vi "Esis_PitchRollAng_PitchRollYawRate_Set_Get.vi"(0 "message handle in1":u64, 1 "message handle in 2":u64, 2 "message handle in 3":u64, 3 "message handle in 4":u64, 4 "message handle in 5":u64, 5 "Esis Pitch Angle":dbl, 6 "Esis Roll Angle":dbl, 7 "Esis Pitch Rate":dbl, 8 "Esis Roll Rate":dbl, 9 "Esis Yaw Rate":dbl, 10 "Esis Pitch Angle Valid":u16, 11 "Esis Roll Angle Valid":u16, 12 "Esis Pitch Rate Valid":u16, 13 "Esis Roll Rate Valid":u16, 14 "Esis Yaw Rate Valid":u16, 15 "error in (no error)":errorcluster) -> (16 "Esis Yaw Rate Value NEW":u32 format="%08b", 18 "Esis Roll Rate Range Message":string, 19 "Esis Yaw Rate Range Message":string, 20 "Esis Pitch Angle Value NEW":u32 format="%08b", 21 "Esis Roll Angle Value NEW":u32 format="%08b", 22 "Esis Pitch Rate Value NEW":u32 format="%08b", 23 "Esis Roll Rate Value NEW":u32 format="%08b", 24 "Esis Pitch Angle Range Message":string, 25 "Esis Roll Angle Range Message":string, 26 "Esis Pitch Rate Range Message":string, 27 "error out":errorcluster)   [LabVIEW 2023]
uses:
  <instrlib>/BTI429Lib/BTI429LV.lvlib
  <instrlib>/BTI429Lib/Private/Utility/Set BNR Data.vi
  <instrlib>/BTI429Lib/Private/Utility/Get BNR Data.vi
  <instrlib>/BTI429Lib/Private/Utility/Set BNR SSM.vi
panel:
  out "Esis Yaw Rate Value OLD":u32 format="%08b"
  out "Esis Roll Rate Value OLD":u32 format="%08b"
  out "Esis Pitch Rate Value OLD":u32 format="%08b"
  out "Esis Roll Angle Value OLD":u32 format="%.0b"
  out "Esis Pitch Angle Value OLD":u32 format="%.0b"
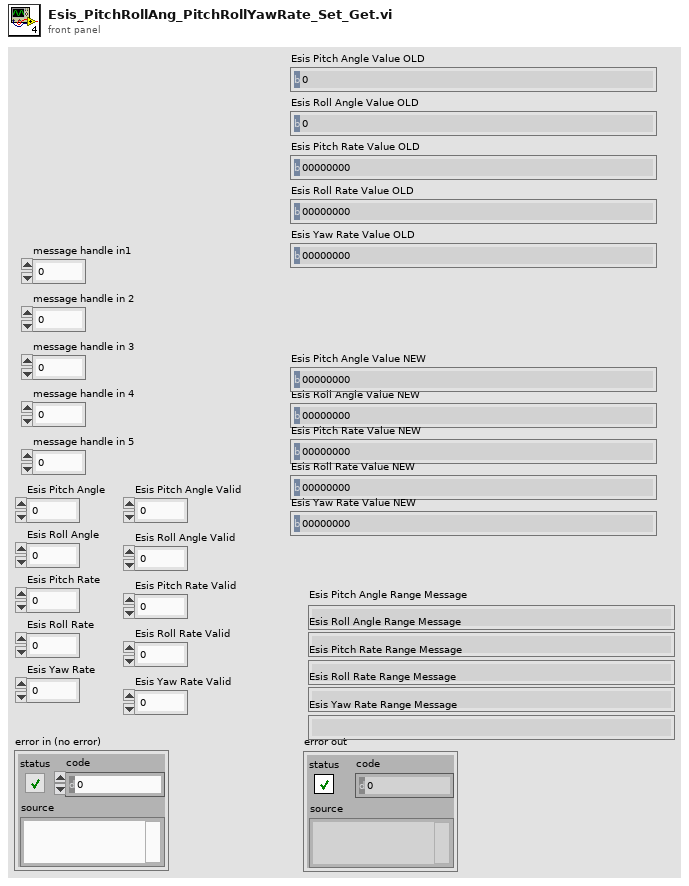
[diagram p1: front panel]
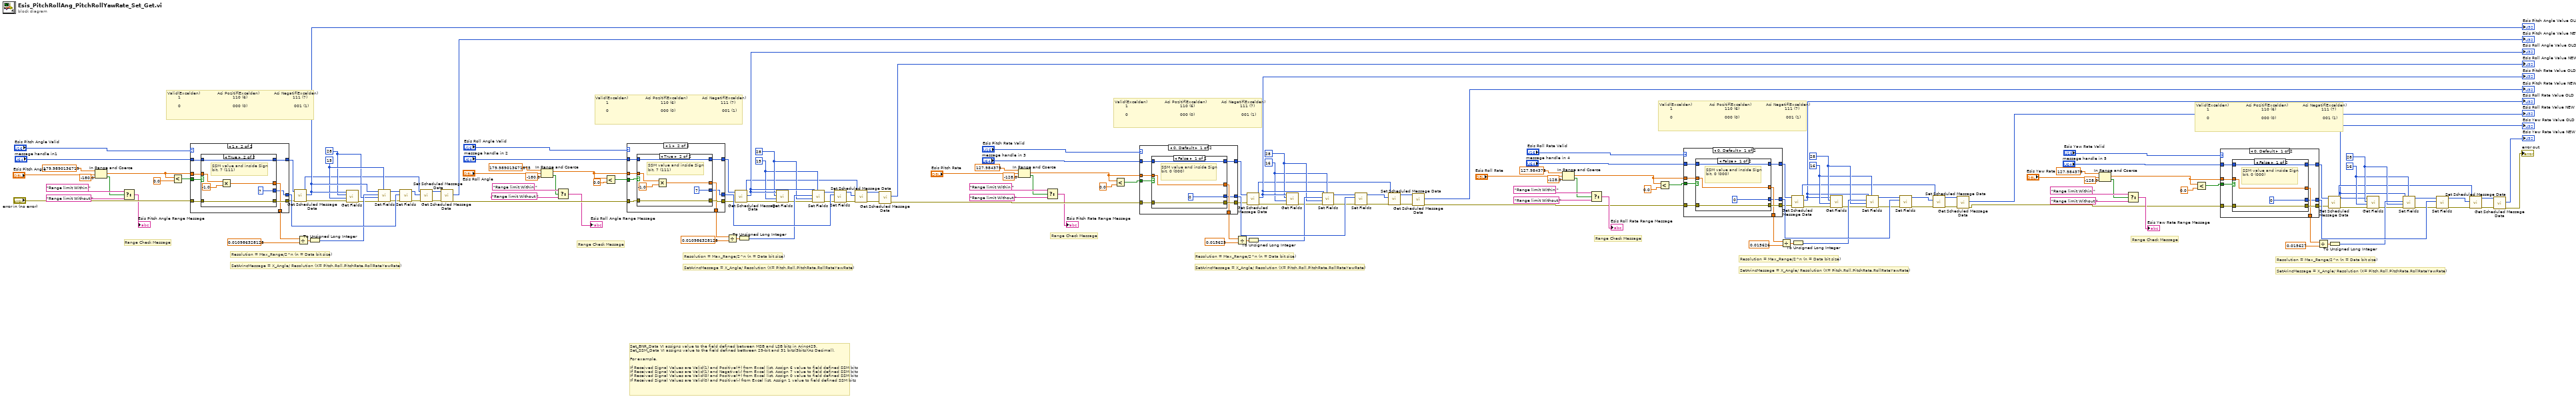
[diagram p0: block diagram]
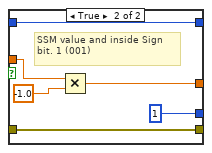
[diagram p2: hidden frame]
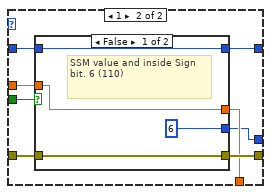
[diagram p3: hidden frame]
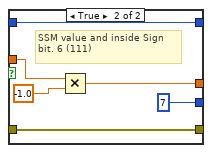
[diagram p4: hidden frame]
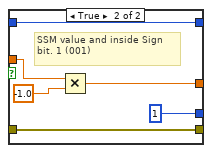
[diagram p5: hidden frame]
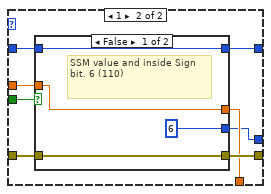
[diagram p6: hidden frame]
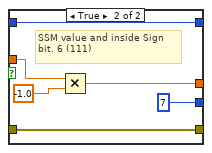
[diagram p7: hidden frame]
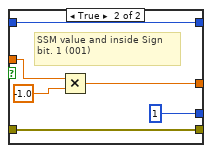
[diagram p8: hidden frame]
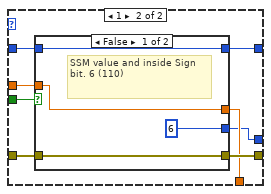
[diagram p9: hidden frame]
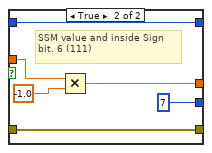
[diagram p10: hidden frame]
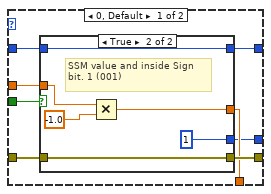
[diagram p11: hidden frame]
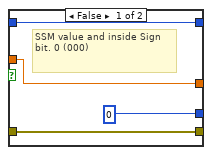
[diagram p12: hidden frame]
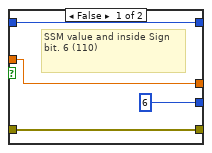
[diagram p13: hidden frame]
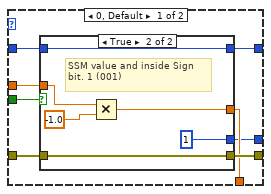
[diagram p14: hidden frame]
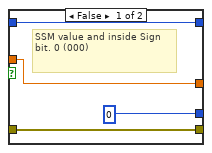
[diagram p15: hidden frame]
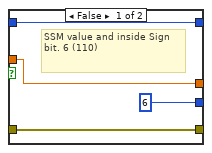
[diagram p16: hidden frame]
diagram:
  w13 = u16 28 ("most significant bit")
  w12 = u16 16 ("least significant bit")
  w43 = u16 28 ("most significant bit")
  w42 = u16 16 ("least significant bit")
  w73 = u16 28 ("most significant bit")
  w72 = u16 16 ("least significant bit")
  w93 = u16 28 ("most significant bit")
  w92 = u16 15 ("least significant bit")
  w84 = u16 28 ("most significant bit")
  w85 = u16 15 ("least significant bit")
  # "Range Check Message"
  # "SetArincMessage = X_Angle/ Resolution (X= Pitch,Roll,PitchRate,RollRateYawRate)"
  # "Resolution = Max_Range/2^n (n = Data bit size)"
  # "Valid(Excelden)             Aci Pozitif(Excelden)           Aci Negatif(Excelden) \n        1                                       110 (6)                                  111 (7)\n\n        0                                       000 (0)                                   001 (1)"
  # "Range Check Message"
  # "SetArincMessage = X_Angle/ Resolution (X= Pitch,Roll,PitchRate,RollRateYawRate)"
  # "Resolution = Max_Range/2^n (n = Data bit size)"
  # "Valid(Excelden)             Aci Pozitif(Excelden)           Aci Negatif(Excelden) \n        1                                       110 (6)                                  111 (7)\n\n        0                                       000 (0)                                   001 (1)"
  # "Range Check Message"
  # "SetArincMessage = X_Angle/ Resolution (X= Pitch,Roll,PitchRate,RollRateYawRate)"
  # "Resolution = Max_Range/2^n (n = Data bit size)"
  # "Range Check Message"
  # "Range Check Message"
  # "SetArincMessage = X_Angle/ Resolution (X= Pitch,Roll,PitchRate,RollRateYawRate)"
  # "Resolution = Max_Range/2^n (n = Data bit size)"
  # "SetArincMessage = X_Angle/ Resolution (X= Pitch,Roll,PitchRate,RollRateYawRate)"
  # "Resolution = Max_Range/2^n (n = Data bit size)"
  # "Set_BNR_Data VI assigns value to the field defined between MSB and LSB bits in Arinc429.\nSet_SSM_Data VI assigns value to the field defined bettween 29-bit and 31 bits(3bits)(As Decimal).\n\nFor example,\n\nIf Received Signal Values are Valid(1) and Positive(+) from Excel list. Assign 6 value to field defined SSM bits\nIf Received Signal Values are Valid(1) and Negative(-) from Excel list. Assign 7 value to field defined SSM bits\nIf Received Signal Values are Valid(0) and Positive(+) from Excel list. Assign 0 value to field defined SSM bits\nIf Received Signal Values are Valid(0) and Positive(-) from Excel list. Assign 1 value to field defined SSM bits"
  # "Valid(Excelden)             Aci Pozitif(Excelden)           Aci Negatif(Excelden) \n        1                                       110 (6)                                  111 (7)\n\n        0                                       000 (0)                                   001 (1)"
  # "Valid(Excelden)             Aci Pozitif(Excelden)           Aci Negatif(Excelden) \n        1                                       110 (6)                                  111 (7)\n\n        0                                       000 (0)                                   001 (1)"
  # "Valid(Excelden)             Aci Pozitif(Excelden)           Aci Negatif(Excelden) \n        1                                       110 (6)                                  111 (7)\n\n        0                                       000 (0)                                   001 (1)"
  n1 = In Range and Coerce(upper limit=179.9890136719, x="Esis Pitch Angle", lower limit=-180.0) -> (coerced(x)=w132:dbl, In Range?=w108:bool)
  n2 = Select(t="Range limit Within ", s=w108, f="Range limit Without ") -> (s? t:f=→"Esis Pitch Angle Range Message":string)
  n3 = Less?(x=w132, y=0.0) -> (x < y?=w133:bool)
  n4 = case shown="1" "Esis Pitch Angle Valid" {
    tunnel: [w173 w192] -> w134
    tunnel: [w171 w191] -> w129
    tunnel: "error in (no error)" -> [w174 w190]
    tunnel: "message handle in1" -> [w172 w189]
    tunnel: w133 -> [w167 w188]
    tunnel: [w169 w187] -> w131
    tunnel: w132 -> [w170 w186]
    tunnel: [w168 w185] -> w139
    frame 0, Default {
      n5 = case shown="True" w167 {
        tunnel: w170 -> [w178 w180]
        tunnel: [w178 w183] -> w169
        tunnel: w172 -> [w177 w182]
        tunnel: w174 -> [w176 w181]
        tunnel: [w177 w182] -> w171
        tunnel: [w176 w181] -> w173
        tunnel: [u16 0 ("value") u16 1 ("value")] -> w168
        frame False {
          # "SSM value and inside Sign bit. 0 (000)"
        }
        frame True {
          # "SSM value and inside Sign bit. 1 (001)"
          n6 = Multiply(x=w180, y=-1.0) -> (x*y=w183:dbl)
        }
      }
    }
    frame 1 {
      n7 = case shown="True" w188 {
        tunnel: w186 -> [w196 w201]
        tunnel: [w196 w200] -> w187
        tunnel: w189 -> [w195 w199]
        tunnel: w190 -> [w194 w198]
        tunnel: [w195 w199] -> w191
        tunnel: [w194 w198] -> w192
        tunnel: [u16 6 ("value") u16 7 ("value")] -> w185
        frame False {
          # "SSM value and inside Sign bit. 6 (110)"
        }
        frame True {
          # "SSM value and inside Sign bit. 7 (111)"
          n8 = Multiply(x=w201, y=-1.0) -> (x*y=w200:dbl)
        }
      }
    }
  }
  n9 = call <instrlib>:"Get Scheduled Message Data.vi"("error in (no error)"=w134, "message handle in"=w129) -> ("error out"=w81:errorcluster, "value"=w99:u32, "message handle out"=w83:u64)  [unwired: 7 in]
  "Esis Pitch Angle Value OLD" <- w99
  n10 = Divide(x=w131, y=0.010986328125) -> (x/y=w88:dbl)
  n11 = To Unsigned Long Integer(number=w88) -> (unsigned 32bit integer=w94:u32)
  n12 = call-poly <instrlib>:"Get Fields.vi"("error in (no error)"=w81, "least significant bit"=w85, "most significant bit"=w84, "message"=w99) -> ("error out"=w82:errorcluster)  [unwired: 6 in, 1 out]
  n13 = call-poly <instrlib>:"Set Fields.vi"("least significant bit"=w85, "error in (no error)"=w82, "most significant bit"=w84, "value"=w94, "message"=w99) -> ("error out"=w135:errorcluster, "message out"=w138:u32)  [unwired: 5 in]
  n14 = call-poly <instrlib>:"Set Fields.vi"("error in (no error)"=w135, "value"=w139, "message"=w138) -> ("error out"=w136:errorcluster, "message out"=w137:u32)  [unwired: 7 in]
  n15 = call <instrlib>:"Set Scheduled Message Data.vi"("error in (no error)"=w136, "value"=w137, "message handle in"=w83) -> ("error out"=w104:errorcluster, "message handle out"=w105:u64)  [unwired: 7 in]
  n16 = call <instrlib>:"Get Scheduled Message Data.vi"("error in (no error)"=w104, "message handle in"=w105) -> ("error out"=w143:errorcluster, "value"=→"Esis Pitch Angle Value NEW":u32)  [unwired: 7 in, 1 out]
  n17 = In Range and Coerce(upper limit=179.989013671875, x="Esis Roll Angle", lower limit=-180.0) -> (coerced(x)=w141:dbl, In Range?=w115:bool)
  n18 = Select(t="Range limit Within ", s=w115, f="Range limit Without ") -> (s? t:f=→"Esis Roll Angle Range Message":string)
  n19 = Less?(x=w141, y=0.0) -> (x < y?=w142:bool)
  n20 = case shown="1" "Esis Roll Angle Valid" {
    tunnel: [w209 w228] -> w145
    tunnel: [w205 w227] -> w146
    tunnel: w143 -> [w210 w226]
    tunnel: "message handle in 2" -> [w204 w225]
    tunnel: w142 -> [w203 w224]
    tunnel: [w207 w223] -> w144
    tunnel: w141 -> [w208 w222]
    tunnel: [w206 w221] -> w151
    frame 0, Default {
      n21 = case shown="True" w203 {
        tunnel: w208 -> [w214 w216]
        tunnel: [w214 w219] -> w207
        tunnel: w204 -> [w213 w218]
        tunnel: w210 -> [w212 w217]
        tunnel: [w213 w218] -> w205
        tunnel: [w212 w217] -> w209
        tunnel: [u16 0 ("value") u16 1 ("value")] -> w206
        frame False {
          # "SSM value and inside Sign bit. 0 (000)"
        }
        frame True {
          # "SSM value and inside Sign bit. 1 (001)"
          n22 = Multiply(x=w216, y=-1.0) -> (x*y=w219:dbl)
        }
      }
    }
    frame 1 {
      n23 = case shown="True" w224 {
        tunnel: w222 -> [w232 w237]
        tunnel: [w232 w236] -> w223
        tunnel: w225 -> [w231 w235]
        tunnel: w226 -> [w230 w234]
        tunnel: [w231 w235] -> w227
        tunnel: [w230 w234] -> w228
        tunnel: [u16 6 ("value") u16 7 ("value")] -> w221
        frame False {
          # "SSM value and inside Sign bit. 6 (110)"
        }
        frame True {
          # "SSM value and inside Sign bit. 7 (111)"
          n24 = Multiply(x=w237, y=-1.0) -> (x*y=w236:dbl)
        }
      }
    }
  }
  n25 = Divide(x=w144, y=0.010986328125) -> (x/y=w97:dbl)
  n26 = call <instrlib>:"Get Scheduled Message Data.vi"("error in (no error)"=w145, "message handle in"=w146) -> ("error out"=w90:errorcluster, "value"=w100:u32, "message handle out"=w89:u64)  [unwired: 7 in]
  "Esis Roll Angle Value OLD" <- w100
  n27 = To Unsigned Long Integer(number=w97) -> (unsigned 32bit integer=w98:u32)
  n28 = call-poly <instrlib>:"Get Fields.vi"("error in (no error)"=w90, "least significant bit"=w92, "most significant bit"=w93, "message"=w100) -> ("error out"=w91:errorcluster)  [unwired: 6 in, 1 out]
  n29 = call-poly <instrlib>:"Set Fields.vi"("least significant bit"=w92, "error in (no error)"=w91, "most significant bit"=w93, "value"=w98, "message"=w100) -> ("error out"=w147:errorcluster, "message out"=w150:u32)  [unwired: 5 in]
  n30 = call-poly <instrlib>:"Set Fields.vi"("error in (no error)"=w147, "value"=w151, "message"=w150) -> ("error out"=w148:errorcluster, "message out"=w149:u32)  [unwired: 7 in]
  n31 = call <instrlib>:"Set Scheduled Message Data.vi"("error in (no error)"=w148, "value"=w149, "message handle in"=w89) -> ("error out"=w101:errorcluster, "message handle out"=w102:u64)  [unwired: 7 in]
  n32 = call <instrlib>:"Get Scheduled Message Data.vi"("error in (no error)"=w101, "message handle in"=w102) -> ("error out"=w152:errorcluster, "value"=→"Esis Roll Angle Value NEW":u32)  [unwired: 7 in, 1 out]
  n33 = In Range and Coerce(upper limit=127.984375, x="Esis Pitch Rate", lower limit=-128.0) -> (coerced(x)=w154:dbl, In Range?=w122:bool)
  n34 = Select(t="Range limit Within ", s=w122, f="Range limit Without ") -> (s? t:f=→"Esis Pitch Rate Range Message":string)
  n35 = Less?(x=w154, y=0.0) -> (x < y?=w153:bool)
  n36 = case shown="0, Default" "Esis Pitch Rate Valid" {
    tunnel: [w245 w264] -> w157
    tunnel: [w241 w263] -> w156
    tunnel: w152 -> [w246 w262]
    tunnel: "message handle in 3" -> [w240 w261]
    tunnel: w153 -> [w239 w260]
    tunnel: [w243 w259] -> w158
    tunnel: w154 -> [w244 w258]
    tunnel: [w242 w257] -> w163
    frame 0, Default {
      n37 = case shown="False" w239 {
        tunnel: w244 -> [w250 w252]
        tunnel: [w250 w255] -> w243
        tunnel: w240 -> [w249 w254]
        tunnel: w246 -> [w248 w253]
        tunnel: [w249 w254] -> w241
        tunnel: [w248 w253] -> w245
        tunnel: [u16 0 ("value") u16 1 ("value")] -> w242
        frame False {
          # "SSM value and inside Sign bit. 0 (000)"
        }
        frame True {
          # "SSM value and inside Sign bit. 1 (001)"
          n38 = Multiply(x=w252, y=-1.0) -> (x*y=w255:dbl)
        }
      }
    }
    frame 1 {
      n39 = case shown="False" w260 {
        tunnel: w258 -> [w268 w273]
        tunnel: [w268 w272] -> w259
        tunnel: w261 -> [w267 w271]
        tunnel: w262 -> [w266 w270]
        tunnel: [w267 w271] -> w263
        tunnel: [w266 w270] -> w264
        tunnel: [u16 6 ("value") u16 7 ("value")] -> w257
        frame False {
          # "SSM value and inside Sign bit. 6 (110)"
        }
        frame True {
          # "SSM value and inside Sign bit. 6 (111)"
          n40 = Multiply(x=w273, y=-1.0) -> (x*y=w272:dbl)
        }
      }
    }
  }
  n41 = Divide(x=w158, y=0.015625) -> (x/y=w76:dbl)
  n42 = call <instrlib>:"Get Scheduled Message Data.vi"("error in (no error)"=w157, "message handle in"=w156) -> ("error out"=w70:errorcluster, "value"=w78:u32, "message handle out"=w69:u64)  [unwired: 7 in]
  "Esis Pitch Rate Value OLD" <- w78
  n43 = To Unsigned Long Integer(number=w76) -> (unsigned 32bit integer=w77:u32)
  n44 = call-poly <instrlib>:"Get Fields.vi"("error in (no error)"=w70, "least significant bit"=w72, "most significant bit"=w73, "message"=w78) -> ("error out"=w71:errorcluster)  [unwired: 6 in, 1 out]
  n45 = call-poly <instrlib>:"Set Fields.vi"("least significant bit"=w72, "error in (no error)"=w71, "most significant bit"=w73, "value"=w77, "message"=w78) -> ("error out"=w159:errorcluster, "message out"=w162:u32)  [unwired: 5 in]
  n46 = call-poly <instrlib>:"Set Fields.vi"("error in (no error)"=w159, "value"=w163, "message"=w162) -> ("error out"=w160:errorcluster, "message out"=w161:u32)  [unwired: 7 in]
  n47 = call <instrlib>:"Set Scheduled Message Data.vi"("error in (no error)"=w160, "value"=w161, "message handle in"=w69) -> ("error out"=w79:errorcluster, "message handle out"=w80:u64)  [unwired: 7 in]
  n48 = call <instrlib>:"Get Scheduled Message Data.vi"("error in (no error)"=w79, "message handle in"=w80) -> ("error out"=w7:errorcluster, "value"=→"Esis Pitch Rate Value NEW":u32)  [unwired: 7 in, 1 out]
  n49 = In Range and Coerce(upper limit=127.984375, x="Esis Roll Rate", lower limit=-128.0) -> (coerced(x)=w58:dbl, In Range?=w51:bool)
  n50 = Select(t="Range limit Within ", s=w51, f="Range limit Without ") -> (s? t:f=→"Esis Roll Rate Range Message":string)
  n51 = Less?(x=w58, y=0.0) -> (x < y?=w57:bool)
  n52 = case shown="0, Default" "Esis Roll Rate Valid" {
    tunnel: [w281 w300] -> w61
    tunnel: [w277 w299] -> w60
    tunnel: w7 -> [w282 w298]
    tunnel: "message handle in 4" -> [w276 w297]
    tunnel: w57 -> [w275 w296]
    tunnel: [w279 w295] -> w62
    tunnel: w58 -> [w280 w294]
    tunnel: [w278 w293] -> w67
    frame 0, Default {
      n53 = case shown="False" w275 {
        tunnel: w280 -> [w286 w288]
        tunnel: [w286 w291] -> w279
        tunnel: w276 -> [w285 w290]
        tunnel: w282 -> [w284 w289]
        tunnel: [w285 w290] -> w277
        tunnel: [w284 w289] -> w281
        tunnel: [u16 0 ("value") u16 1 ("value")] -> w278
        frame False {
          # "SSM value and inside Sign bit. 0 (000)"
        }
        frame True {
          # "SSM value and inside Sign bit. 1 (001)"
          n54 = Multiply(x=w288, y=-1.0) -> (x*y=w291:dbl)
        }
      }
    }
    frame 1 {
      n55 = case shown="False" w296 {
        tunnel: w294 -> [w304 w309]
        tunnel: [w304 w308] -> w295
        tunnel: w297 -> [w303 w307]
        tunnel: w298 -> [w302 w306]
        tunnel: [w303 w307] -> w299
        tunnel: [w302 w306] -> w300
        tunnel: [u16 6 ("value") u16 7 ("value")] -> w293
        frame False {
          # "SSM value and inside Sign bit. 6 (110)"
        }
        frame True {
          # "SSM value and inside Sign bit. 6 (111)"
          n56 = Multiply(x=w309, y=-1.0) -> (x*y=w308:dbl)
        }
      }
    }
  }
  n57 = Divide(x=w62, y=0.015626) -> (x/y=w46:dbl)
  n58 = call <instrlib>:"Get Scheduled Message Data.vi"("error in (no error)"=w61, "message handle in"=w60) -> ("error out"=w40:errorcluster, "value"=w4:u32, "message handle out"=w39:u64)  [unwired: 7 in]
  "Esis Roll Rate Value OLD" <- w4
  n59 = To Unsigned Long Integer(number=w46) -> (unsigned 32bit integer=w47:u32)
  n60 = call-poly <instrlib>:"Get Fields.vi"("error in (no error)"=w40, "least significant bit"=w42, "most significant bit"=w43, "message"=w4) -> ("error out"=w41:errorcluster)  [unwired: 6 in, 1 out]
  n61 = call-poly <instrlib>:"Set Fields.vi"("least significant bit"=w42, "error in (no error)"=w41, "most significant bit"=w43, "value"=w47, "message"=w4) -> ("error out"=w63:errorcluster, "message out"=w66:u32)  [unwired: 5 in]
  n62 = call-poly <instrlib>:"Set Fields.vi"("error in (no error)"=w63, "value"=w67, "message"=w66) -> ("error out"=w64:errorcluster, "message out"=w65:u32)  [unwired: 7 in]
  n63 = call <instrlib>:"Set Scheduled Message Data.vi"("error in (no error)"=w64, "value"=w65, "message handle in"=w39) -> ("error out"=w48:errorcluster, "message handle out"=w49:u64)  [unwired: 7 in]
  n64 = call <instrlib>:"Get Scheduled Message Data.vi"("error in (no error)"=w48, "message handle in"=w49) -> ("error out"=w8:errorcluster, "value"=→"Esis Roll Rate Value NEW":u32)  [unwired: 7 in, 1 out]
  n65 = In Range and Coerce(upper limit=127.984375, x="Esis Yaw Rate", lower limit=-128.0) -> (coerced(x)=w28:dbl, In Range?=w21:bool)
  n66 = Select(t="Range limit Within ", s=w21, f="Range limit Without ") -> (s? t:f=→"Esis Yaw Rate Range Message":string)
  n67 = Less?(x=w28, y=0.0) -> (x < y?=w27:bool)
  n68 = case shown="0, Default" "Esis Yaw Rate Valid" {
    tunnel: [w317 w336] -> w31
    tunnel: [w313 w335] -> w30
    tunnel: w8 -> [w318 w334]
    tunnel: "message handle in 5" -> [w312 w333]
    tunnel: w27 -> [w311 w332]
    tunnel: [w315 w331] -> w32
    tunnel: w28 -> [w316 w330]
    tunnel: [w314 w329] -> w37
    frame 0, Default {
      n69 = case shown="False" w311 {
        tunnel: w316 -> [w322 w324]
        tunnel: [w322 w327] -> w315
        tunnel: w312 -> [w321 w326]
        tunnel: w318 -> [w320 w325]
        tunnel: [w321 w326] -> w313
        tunnel: [w320 w325] -> w317
        tunnel: [u16 0 ("value") u16 1 ("value")] -> w314
        frame False {
          # "SSM value and inside Sign bit. 0 (000)"
        }
        frame True {
          # "SSM value and inside Sign bit. 1 (001)"
          n70 = Multiply(x=w324, y=-1.0) -> (x*y=w327:dbl)
        }
      }
    }
    frame 1 {
      n71 = case shown="False" w332 {
        tunnel: w330 -> [w340 w345]
        tunnel: [w340 w344] -> w331
        tunnel: w333 -> [w339 w343]
        tunnel: w334 -> [w338 w342]
        tunnel: [w339 w343] -> w335
        tunnel: [w338 w342] -> w336
        tunnel: [u16 6 ("value") u16 7 ("value")] -> w329
        frame False {
          # "SSM value and inside Sign bit. 6 (110)"
        }
        frame True {
          # "SSM value and inside Sign bit. 6 (111)"
          n72 = Multiply(x=w345, y=-1.0) -> (x*y=w344:dbl)
        }
      }
    }
  }
  n73 = Divide(x=w32, y=0.015627) -> (x/y=w16:dbl)
  n74 = call <instrlib>:"Get Scheduled Message Data.vi"("error in (no error)"=w31, "message handle in"=w30) -> ("error out"=w10:errorcluster, "value"=w3:u32, "message handle out"=w9:u64)  [unwired: 7 in]
  "Esis Yaw Rate Value OLD" <- w3
  n75 = To Unsigned Long Integer(number=w16) -> (unsigned 32bit integer=w17:u32)
  n76 = call-poly <instrlib>:"Get Fields.vi"("error in (no error)"=w10, "least significant bit"=w12, "most significant bit"=w13, "message"=w3) -> ("error out"=w11:errorcluster)  [unwired: 6 in, 1 out]
  n77 = call-poly <instrlib>:"Set Fields.vi"("least significant bit"=w12, "error in (no error)"=w11, "most significant bit"=w13, "value"=w17, "message"=w3) -> ("error out"=w33:errorcluster, "message out"=w36:u32)  [unwired: 5 in]
  n78 = call-poly <instrlib>:"Set Fields.vi"("error in (no error)"=w33, "value"=w37, "message"=w36) -> ("error out"=w34:errorcluster, "message out"=w35:u32)  [unwired: 7 in]
  n79 = call <instrlib>:"Set Scheduled Message Data.vi"("error in (no error)"=w34, "value"=w35, "message handle in"=w9) -> ("error out"=w18:errorcluster, "message handle out"=w19:u64)  [unwired: 7 in]
  n80 = call <instrlib>:"Get Scheduled Message Data.vi"("error in (no error)"=w18, "message handle in"=w19) -> ("error out"=→"error out":errorcluster, "value"=→"Esis Yaw Rate Value NEW":u32)  [unwired: 7 in, 1 out]
